vi "Search to -From.vi"(5 "Enable":bool[](array[boolean])=[FALSE, FALSE, FALSE, FALSE, FALSE, FALSE, FALSE, FALSE, FALSE], 7 "Selection":string[](array[string])=[" and MODELNAME='", " and PARTNAME='", "and PARTNO='", "and SYHC='", "and BYHC='", "and SHC='", "and RSB='", "and SPHC='", "and BBC='"], 10 "From date":timestamp format="%<%H:%M:%S\n%d/%m/%y>T", 11 "To Date":timestamp format="%<%H:%M:%S\n%d/%m/%y>T") -> (3 "search dataString":string)   [LabVIEW 2023]
panel:
  out "String":string
  out "search dataString 2":string
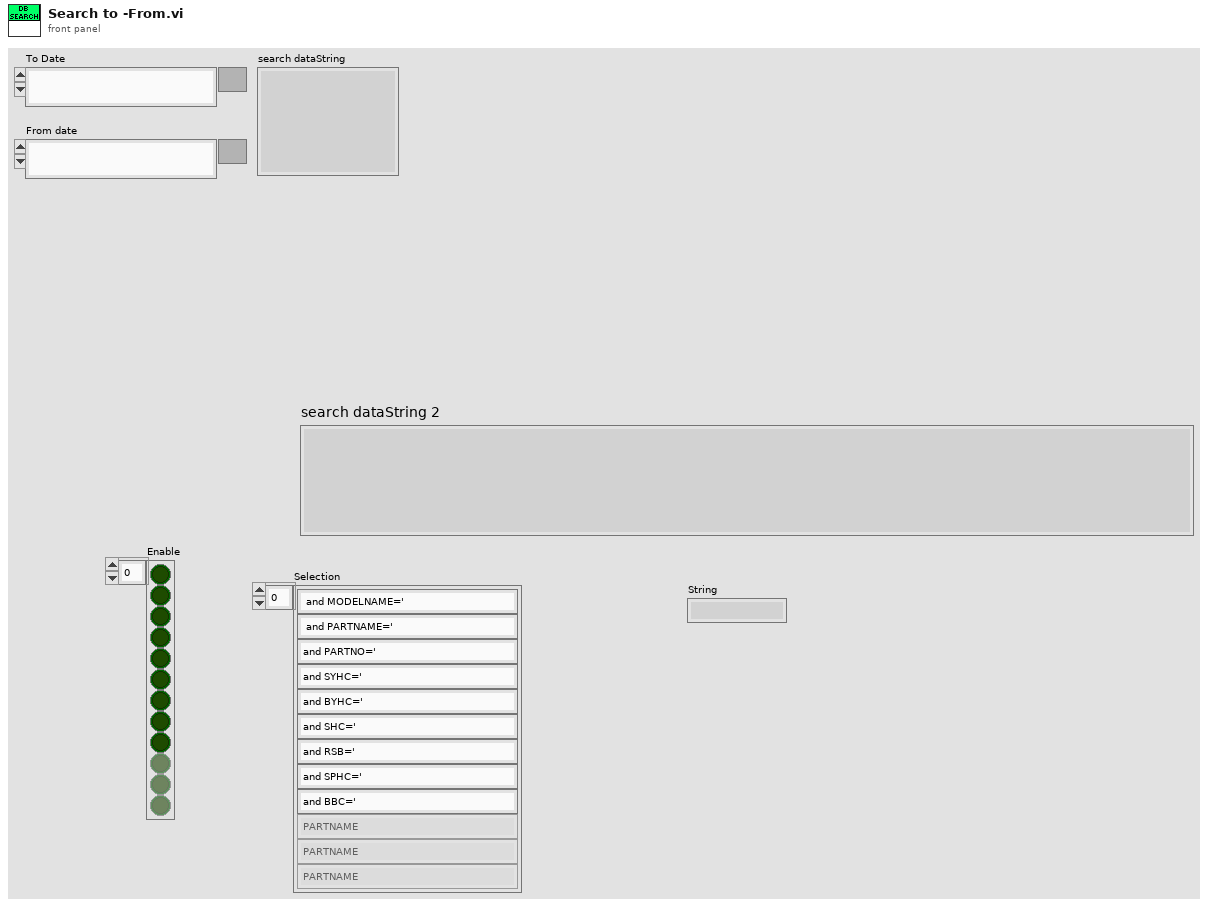
[diagram p1: front panel]
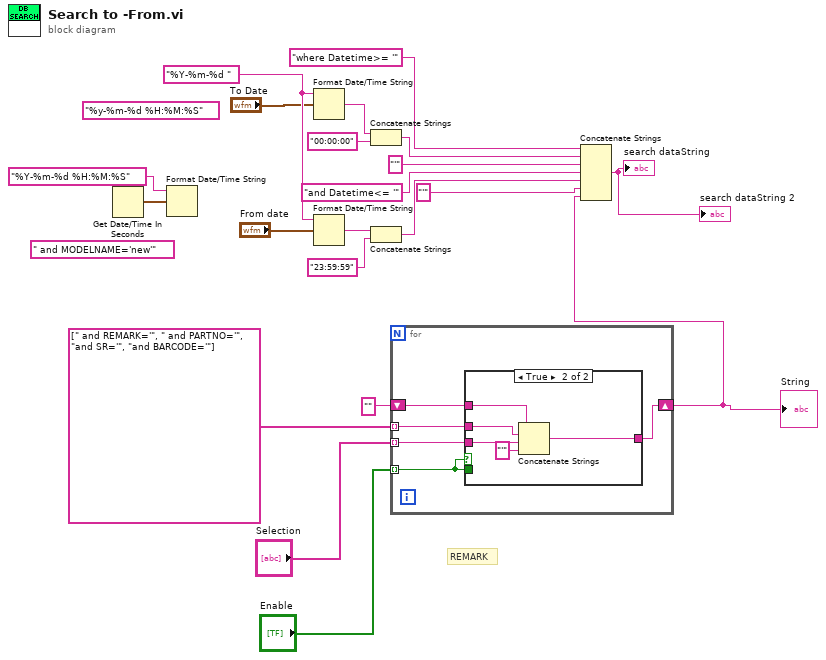
[diagram p0: block diagram]
diagram:
  (unwired) " and MODELNAME='new'" ("string")
  (unwired) "%y-%m-%d %H:%M:%S" ("time format string (%c)")
  w19 = "%Y-%m-%d " ("time format string (%c)")
  # "REMARK"
  n1 = Get Date/Time In Seconds() -> (seconds since 1Jan1904=w1:timestamp)
  n2 = Format Date/Time String(time format string (%c)="%Y-%m-%d %H:%M:%S", seconds (now)=w1) -> ()  [unwired: 1 in, 1 out]
  n3 = Format Date/Time String(time format string (%c)=w19, seconds (now)="To Date") -> (date/time string=w17:string)  [unwired: 1 in]
  n4 = Format Date/Time String(time format string (%c)=w19, seconds (now)="From date") -> (date/time string=w20:string)  [unwired: 1 in]
  n5 = Concatenate Strings(w17, "00:00:00" ("time format string (%c)")) -> (w14:string)
  n6 = Concatenate Strings(w20, "23:59:59" ("time format string (%c)")) -> (w13:string)
  n7 = for {
    tunnel: string[] [" and REMARK='", " and PARTNO='", "and SR='", "and BARCODE='"] -> [w26] mode=indexing
    shift-right: [w22] -> w3
    shift-left: "" -> [w24]
    tunnel: "Enable" -> [w25] mode=indexing
    tunnel: "Selection" -> [w23] mode=indexing
    n8 = case shown="True" w25 {
      tunnel: w26 -> [_ w32]
      tunnel: w25 -> [_ _]
      tunnel: w24 -> [w27 w31]
      tunnel: w23 -> [_ w30]
      tunnel: [w27 w28] -> w22
      frame False {
      }
      frame True {
        n9 = Concatenate Strings(w31, w32, w30, "'" ("string")) -> (w28:string)
      }
    }
  }
  "String" <- w3
  n10 = Concatenate Strings("where Datetime>= '" ("condition"), w14, "'" ("User Name"), "and Datetime<= '" ("string"), w13, "'" ("string"), w3) -> (→"search dataString" →"search dataString 2":string)
